vi "FPGA-TrapTest-19-08-2016.vi"() -> ()   [LabVIEW 2010]
uses:
  <vilib>/eio/EIONode/EIONode.xnode
  <vilib>/rvi/eio/nirviEIOImplementation/nirviEIOImplementation.xnode
  <vilib>/rvi/eio/common/nirviEmuClasses.ctl
  <vilib>/rvi/eio/common/nirviEmuTemplateMethod_noerrors.vi
panel:
  out "Thermoelement":fxp<+/-,26,5> format="%.23g"
  out "PTStirling":fxp<+/-,26,5> format="%.23g"
  in  "Stirling":bool
  out "PTTrap":fxp<+/-,28,7> format="%.24g"
  in  "stop":bool
  in  "setpoint":fxp<+/-,16,6> format="%.12g"
  in  "Messwerte":i32
  in  "Heizen":bool
  in  "5Van(us)":u16
  in  "Periode(us)":u32
  out "Messwert":fxp<+/-,27,6> format="%.23g"
  in  "Warten(us)":u16
  in  "zwischenMesswerten(us)":u16
  in  "PID gains":T1={"proportional gain (Kc)"=1.0, "integral gain (Kc*Ts/Ti)"=1.66796875, "derivative gain (Kc*Td/Ts)"=0.0} {"proportional gain (Kc)" format="%.11g"; "integral gain (Kc*Ts/Ti)" format="%.11g"; "derivative gain (Kc*Td/Ts)" format="%.11g"}
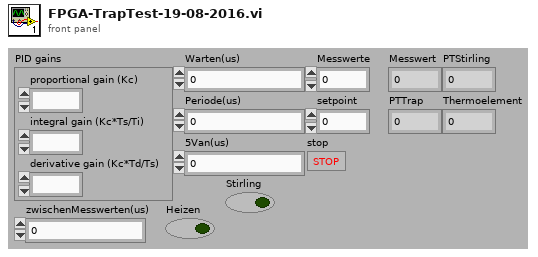
[diagram p1: front panel]
types:
  T1 = cluster{"proportional gain (Kc)":fxp<+/-,16,8>, "integral gain (Kc*Ts/Ti)":fxp<+/-,16,8>, "derivative gain (Kc*Td/Ts)":fxp<+/-,16,8>}
  T2 = typedef "nirviEmuClasses.ctl" = enum16{"IO Read", "IO Write", "Method", "Property Read", "Property Write"}
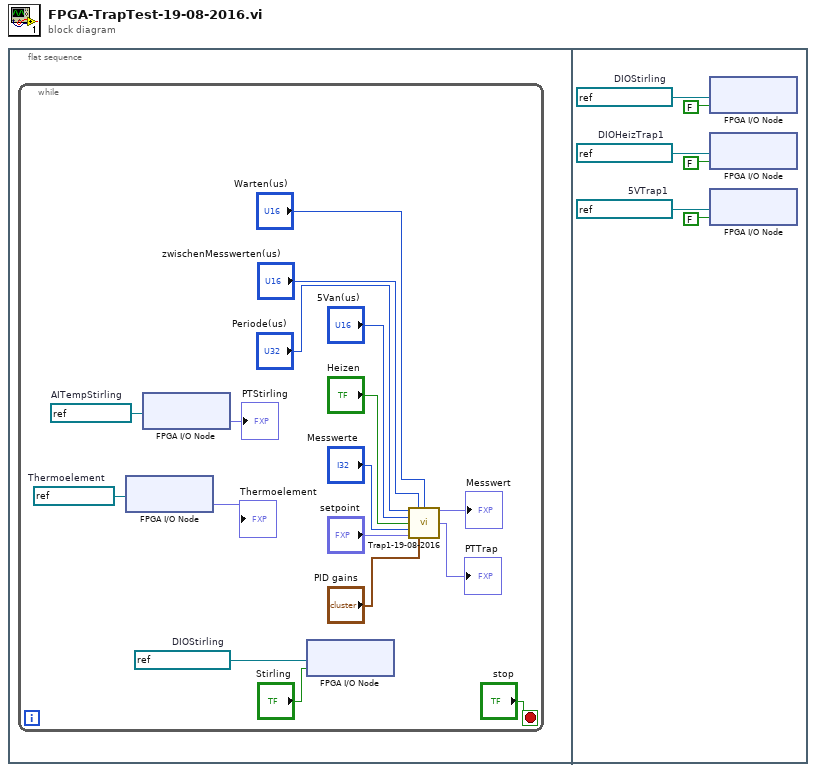
[diagram p0: block diagram]
diagram:
  n1 = flat-sequence {
    frame #0 {
      n2 = while {
        stop <- "stop" stop-if-true
        w2 = refnum<k21> "Mod1/AI3"  # Thermoelement
        w5 = refnum<k21> "Mod1/AI2"  # AITempStirling
        w7 = refnum<k21> "Mod6/DIO12"  # DIOStirling
        n3 = xnode "FPGA I/O Node"("FPGA I/O In"=w2) -> ("I/O Item"=→"Thermoelement":fxp<+/-,26,5>)  [unwired: 1 out]
        n4 = xnode "FPGA I/O Node"("FPGA I/O In"=w5) -> ("I/O Item"=→"PTStirling":fxp<+/-,26,5>)  [unwired: 1 out]
        n5 = xnode "FPGA I/O Node"("I/O Item"="Stirling", "FPGA I/O In"=w7) -> ()  [unwired: 1 out]
        n6 = call "Trap1-19-08-2016.vi"("Periode(us)"="Periode(us)", "zwischenMesswerten(us)"="zwischenMesswerten(us)", "Warten(us)"="Warten(us)", "5Van(us)"="5Van(us)", "Heizen"="Heizen", "Messwerte"="Messwerte", "setpoint"="setpoint", "PID gains"="PID gains") -> ("Messwert"=→"Messwert":fxp<+/-,27,6>, "PTTrap"=→"PTTrap":fxp<+/-,28,7>)  [unwired: 6 in]
      }
    }
    frame #1 {
      w68 = refnum<k21> "Mod6/DIO12"  # DIOStirling
      w70 = refnum<k21> "Mod6/DIO19"  # DIOHeizTrap1
      w72 = refnum<k21> "Mod6/DIO21"  # 5VTrap1
      n7 = xnode "FPGA I/O Node"("I/O Item"=FALSE, "FPGA I/O In"=w68) -> ()  [unwired: 1 out]
      n8 = xnode "FPGA I/O Node"("I/O Item"=FALSE, "FPGA I/O In"=w70) -> ()  [unwired: 1 out]
      n9 = xnode "FPGA I/O Node"("I/O Item"=FALSE, "FPGA I/O In"=w72) -> ()  [unwired: 1 out]
    }
  }
